vi "Main.vi"() -> ()   [LabVIEW 2015]
uses:
  <vilib>/myRIO/Instrument Drivers/Onboard IO/UART/typedef/VISA Configuration.ctl
  <vilib>/Instr/_visa.llb/VISA Configure Serial Port (Instr).vi
  <vilib>/myRIO/Express VI/Onboard IO/UART/UART Express VI.xnode
  <vilib>/myRIO/Instrument Drivers/Onboard IO/UART/UART.lvlib
panel:
  out "Voltage":i16(knob) scale=0.0..5.0
  out "Distance":i16(slide) scale=15.0..50.0
  out "Temperature":i16(knob) scale=20.0..40.0
  in  "stop":bool
  # "The VI commmunicates with Arduino via serial communication and sending three different commands.\nThe commands trigger the reading of random variables: temperature, distance and voltage."
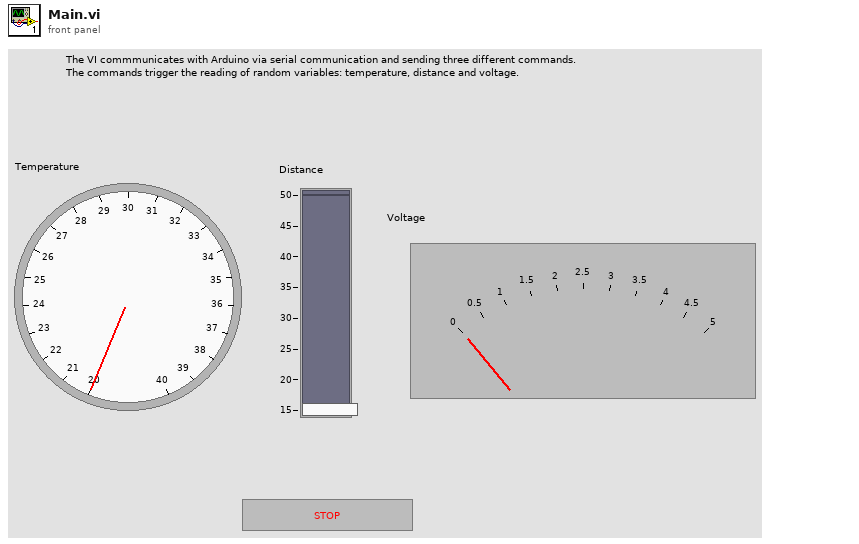
[diagram p1: front panel]
types:
  T1 = typedef "UART.lvlib/VISA Configuration.ctl" = cluster{"baud rate (9600)":u32, "data bits (8)":u16, "parity (0:none)":enum16{"None", "Odd", "Even", "Mark", "Space"}, "stop bits (10: 1 bit)":u16, "flow control (0:none)":u16, "termination char\n(0xA = '\\n' = LF) ":u8, "Enable Termination\nChar (T)":bool, "timeout (10sec)":u32}
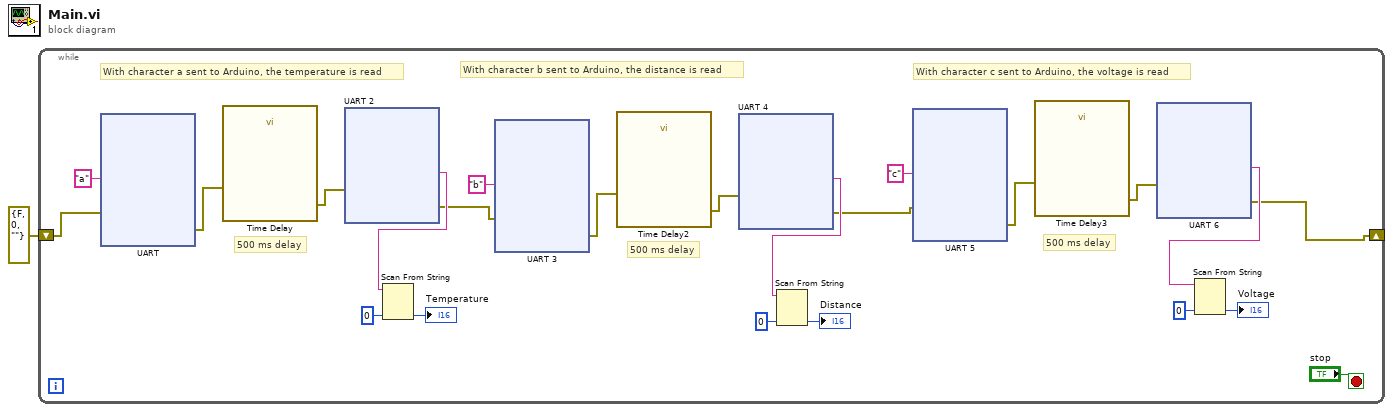
[diagram p0: block diagram]
diagram:
  n1 = while {
    shift-right: [w2] -> _
    shift-left: errorcluster {"status"=FALSE, "code"=0, "source"=""} ("error out") -> [w20]
    stop <- "stop" stop-if-true
    # "500 ms delay"
    # "500 ms delay"
    # "500 ms delay"
    # "With character c sent to Arduino, the voltage is read"
    # "With character b sent to Arduino, the distance is read"
    # "With character a sent to Arduino, the temperature is read"
    n2 = xnode "UART"("Characters to Write"="a", "error in (no error)"=w20) -> ("error out"=w22:errorcluster)  [unwired: 1 out]
    n3 = call "Time Delay"("error in (no error)"=w22) -> ("error out"=w21:errorcluster)  [unwired: 10 in]
    n4 = xnode "UART 2"("error in (no error)"=w21) -> ("Characters Read"=w19:string, "error out"=w6:errorcluster)
    n5 = Scan From String "Scan From String"(input string=w19, default 1=i16 0 ("default value 1")) -> (output 1=→"Temperature":i16)  [unwired: 3 in, 3 out]
    n6 = xnode "UART 3"("Characters to Write"="b", "error in (no error)"=w6) -> ("error out"=w12:errorcluster)  [unwired: 1 out]
    n7 = call "Time Delay2"("error in (no error)"=w12) -> ("error out"=w13:errorcluster)  [unwired: 10 in]
    n8 = xnode "UART 4"("error in (no error)"=w13) -> ("Characters Read"=w14:string, "error out"=w5:errorcluster)
    n9 = Scan From String "Scan From String"(input string=w14, default 1=i16 0 ("default value 1")) -> (output 1=→"Distance":i16)  [unwired: 3 in, 3 out]
    n10 = xnode "UART 5"("Characters to Write"="c", "error in (no error)"=w5) -> ("error out"=w10:errorcluster)  [unwired: 1 out]
    n11 = call "Time Delay3"("error in (no error)"=w10) -> ("error out"=w9:errorcluster)  [unwired: 10 in]
    n12 = xnode "UART 6"("error in (no error)"=w9) -> ("Characters Read"=w3:string, "error out"=w2:errorcluster)
    n13 = Scan From String "Scan From String"(input string=w3, default 1=i16 0 ("default value 1")) -> (output 1=→"Voltage":i16)  [unwired: 3 in, 3 out]
  }
